vi "T1_M.vi"(0 "a":dbl=6378137.0 format="%_20g", 2 "b":dbl=6356752.3142 format="%_20g", 3 "fi":dbl=6356752.314 format="%_20g") -> (7 "T1_M":dbl format="%.20g")   [LabVIEW 2015, in "Biblioteka moduł map v3.lvlib" / "Konwersja wsp.lvlib" / "UTM.lvlib" / "Konwersja na UTM.lvlib"]
doc: "Współczynnik wzoru na konwersję na UTM."
uses:
  Konwersja na UTM.lvlib
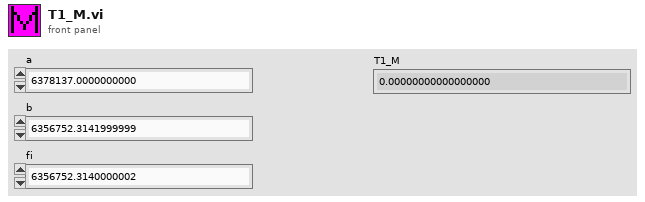
[diagram p1: front panel]
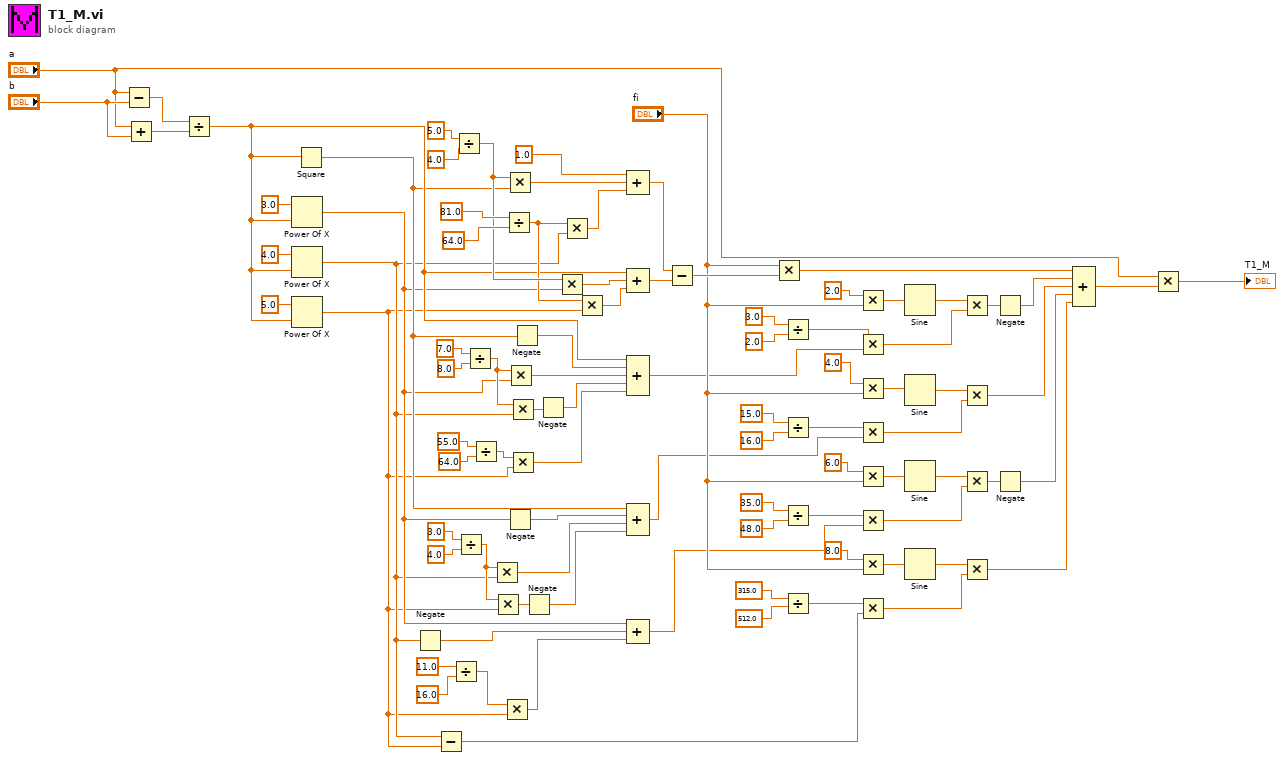
[diagram p0: block diagram]
diagram:
  n1 = Subtract(x="a", y="b") -> (x-y=w90:dbl)
  n2 = Add(x="a", y="b") -> (x+y=w89:dbl)
  n3 = Divide(x=w90, y=w89) -> (x/y=w14:dbl)
  n4 = Power Of X(1:w14, 2:3.0 ("y")) -> (0:w9:dbl)
  n5 = Power Of X(1:w14, 2:4.0 ("y")) -> (0:w8:dbl)
  n6 = Power Of X(1:w14, 2:5.0 ("y")) -> (0:w4:dbl)
  n7 = Square(x=w14) -> (x^2=w12:dbl)
  n8 = Negate(x=w8) -> (-x=w32:dbl)
  n9 = Subtract(x=w8, y=w4) -> (x-y=w33:dbl)
  n10 = Divide(x=11.0, y=16.0) -> (x/y=w31:dbl)
  n11 = Divide(x=5.0, y=4.0) -> (x/y=w78:dbl)
  n12 = Divide(x=3.0, y=4.0) -> (x/y=w23:dbl)
  n13 = Divide(x=7.0, y=8.0) -> (x/y=w11:dbl)
  n14 = Divide(x=55.0, y=64.0) -> (x/y=w5:dbl)
  n15 = Multiply(x=w23, y=w8) -> (x*y=w21:dbl)
  n16 = Multiply(x=w23, y=w4) -> (x*y=w22:dbl)
  n17 = Multiply(x=w31, y=w4) -> (x*y=w28:dbl)
  n18 = Divide(x=81.0, y=64.0) -> (x/y=w74:dbl)
  n19 = Multiply(x=w78, y=w12) -> (x*y=w84:dbl)
  n20 = Negate(x=w9) -> (-x=w26:dbl)
  n21 = Multiply(x=w11, y=w9) -> (x*y=w6:dbl)
  n22 = Multiply(x=w11, y=w8) -> (x*y=w10:dbl)
  n23 = Multiply(x=w5, y=w4) -> (x*y=w3:dbl)
  n24 = Negate(x=w12) -> (-x=w13:dbl)
  n25 = Negate(x=w22) -> (-x=w20:dbl)
  n26 = Negate(x=w10) -> (-x=w7:dbl)
  n27 = Multiply(x=w78, y=w9) -> (x*y=w76:dbl)
  n28 = Multiply(x=w74, y=w8) -> (x*y=w80:dbl)
  n29 = Multiply(x=w74, y=w4) -> (x*y=w73:dbl)
  n30 = Compound Arithmetic op=ADD(1.0 ("value"), w84, w80) -> (w88:dbl)
  n31 = Compound Arithmetic op=ADD(w14, w76, w73) -> (w87:dbl)
  n32 = Compound Arithmetic op=ADD(w14, w13, w6, w7, w3) -> (w2:dbl)
  n33 = Compound Arithmetic op=ADD(w12, w26, w21, w20) -> (w19:dbl)
  n34 = Compound Arithmetic op=ADD(w9, w32, w28) -> (w27:dbl)
  n35 = Subtract(x=w88, y=w87) -> (x-y=w72:dbl)
  n36 = Multiply(x="fi", y=w72) -> (x*y=w70:dbl)
  n37 = Divide(x=3.0, y=2.0) -> (x/y=w43:dbl)
  n38 = Divide(x=15.0, y=16.0) -> (x/y=w44:dbl)
  n39 = Divide(x=35.0, y=48.0) -> (x/y=w48:dbl)
  n40 = Divide(x=315.0, y=512.0) -> (x/y=w49:dbl)
  n41 = Multiply(x=2.0, y="fi") -> (x*y=w55:dbl)
  n42 = Multiply(x=w43, y=w2) -> (x*y=w42:dbl)
  n43 = Multiply(x=4.0, y="fi") -> (x*y=w56:dbl)
  n44 = Multiply(x=w44, y=w19) -> (x*y=w45:dbl)
  n45 = Multiply(x=6.0, y="fi") -> (x*y=w58:dbl)
  n46 = Multiply(x=w48, y=w27) -> (x*y=w47:dbl)
  n47 = Multiply(x=8.0, y="fi") -> (x*y=w57:dbl)
  n48 = Multiply(x=w49, y=w33) -> (x*y=w46:dbl)
  n49 = Sine(x=w55) -> (sin(x)=w62:dbl)
  n50 = Sine(x=w56) -> (sin(x)=w59:dbl)
  n51 = Sine(x=w58) -> (sin(x)=w60:dbl)
  n52 = Sine(x=w57) -> (sin(x)=w61:dbl)
  n53 = Multiply(x=w62, y=w42) -> (x*y=w66:dbl)
  n54 = Multiply(x=w59, y=w45) -> (x*y=w65:dbl)
  n55 = Multiply(x=w60, y=w47) -> (x*y=w64:dbl)
  n56 = Multiply(x=w61, y=w46) -> (x*y=w63:dbl)
  n57 = Negate(x=w66) -> (-x=w68:dbl)
  n58 = Negate(x=w64) -> (-x=w67:dbl)
  n59 = Compound Arithmetic op=ADD(w70, w68, w65, w67, w63) -> (w69:dbl)
  n60 = Multiply(x="a", y=w69) -> (x*y=→"T1_M":dbl)
